vi "PI_Image_Scanner_Prepare.vi"(0 "x-Pixel":u16=100, 1 "y-Pixel":u16=100, 3 "Picture size x":dbl=20.0 min=0.1 max=200.0 format="%1.1f um", 4 "Picture size y":dbl=20.0 min=0.1 max=200.0 format="%1.1f um", 7 "Axis":enum32{"x-y", "x-z", "y-z"}(ring), 9 "Scanner Divider":i32) -> (14 "Commandset out":string[](array[string]), 16 "Measurement time / [s]":dbl)   [LabVIEW 2011]
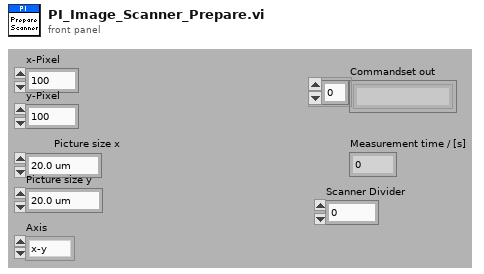
[diagram p1: front panel]
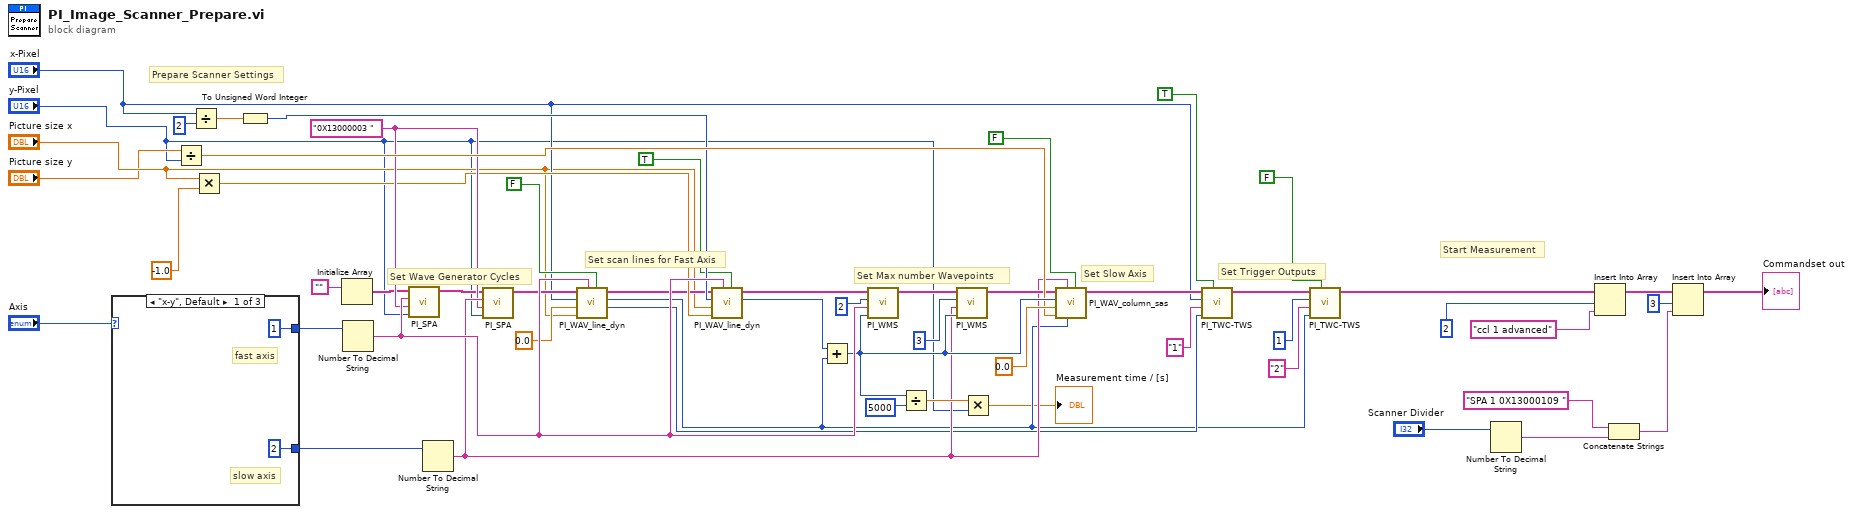
[diagram p0: block diagram]
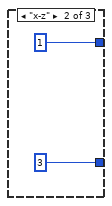
[diagram p2: hidden frame]
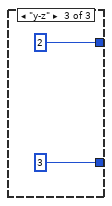
[diagram p3: hidden frame]
diagram:
  w41 = "0X13000003 " ("string")
  # "Start Measurement"
  # "Set Slow Axis"
  # "Set Trigger Outputs"
  # "Set Max number Wavepoints"
  # "Set scan lines for Fast Axis"
  # "Set Wave Generator Cycles"
  # "Prepare Scanner Settings"
  n1 = case shown="\"x-y\", Default" "Axis" {
    tunnel: [1 1 2] -> w27
    tunnel: [2 3 3] -> w28
    frame "x-y", Default {
      # "slow axis"
      # "fast axis"
    }
    frame "x-z" {
    }
    frame "y-z" {
    }
  }
  n2 = Divide(x="Picture size y", y="y-Pixel") -> (x/y=w49:dbl)
  n3 = Divide(x="x-Pixel", y=u16 2) -> (x/y=w33:dbl)
  n4 = Multiply(x="Picture size x", y=-1.0) -> (x*y=w35:dbl)
  n5 = To Unsigned Word Integer(number=w33) -> (unsigned 16bit integer=w34:u16)
  n6 = Initialize Array("") -> (w39:string[])  [unwired: 1 out]
  n7 = Number To Decimal String(number=w27) -> (decimal integer string=w55:string)  [unwired: 1 out]
  n8 = call "PI_SPA.vi"("Value"="y-Pixel", "Register"=w41, "Axis"=w55, "Commandset in"=w39) -> ("Commandset out"=w40:string[])  [unwired: 7 out]
  n9 = Number To Decimal String(number=w28) -> (decimal integer string=w47:string)  [unwired: 1 out]
  n10 = call "PI_SPA.vi"("Value"="y-Pixel", "Register"=w41, "Axis"=w47, "Commandset in"=w40) -> ("Commandset out"=w38:string[])  [unwired: 7 out]
  n11 = call "PI_WAV_line_dyn.vi"("Attach to wav"=FALSE, "Axis Identifier"=w55, "Amplitude / [mu]"="Picture size x", "Startpos / [mu]"=0.0, "Pixel per scan"="x-Pixel", "Commandset in"=w38) -> ("Curve-Start-Pixel"=w24:u16, "Num_Pix"=w17:u16, "Commandset out"=w30:string[])  [unwired: 3 out]
  n12 = call "PI_WAV_line_dyn.vi"("Attach to wav"=TRUE, "Axis Identifier"=w55, "Amplitude / [mu]"=w35, "Startpos / [mu]"="Picture size x", "Pixel per scan"=w34, "Commandset in"=w30) -> ("Num_Pix"=w37:u16, "Commandset out"=w42:string[])  [unwired: 4 out]
  n13 = Add(x=w37, y=w17) -> (x+y=w52:u16)
  n14 = call "PI_WMS.vi"("Pixels to reserve"=w52, "Axis"=w55, "Position / Commandset"=2, "Commandset in"=w42) -> ("Commandset out"=w43:string[])  [unwired: 7 out]
  n15 = Divide(x=w52, y=5000) -> (x/y=w54:dbl)
  n16 = call "PI_WMS.vi"("Pixels to reserve"=w52, "Axis"=w47, "Position / Commandset"=3, "Commandset in"=w43) -> ("Commandset out"=w48:string[])  [unwired: 7 out]
  n17 = Multiply(x=w54, y="y-Pixel") -> (x*y=→"Measurement time / [s]":dbl)
  n18 = call "PI_WAV_column_sas.vi"("Attach to wav"=FALSE, "Steps per Scan-line"=w17, "Axis Identifier"=w47, "Amplitude / [mu]"=w49, "Startpos / [mu]"=0.0, "Pixel per scan"=w52, "Commandset in"=w48) -> ("Commandset out"=w25:string[])  [unwired: 4 out]
  n19 = call "PI_TWC-TWS.vi"("TWC?"=TRUE, "Curve_Start_Pixel"=w24, "Axis Identifier"="1", "Pixel per scan"="x-Pixel", "Commandset in"=w25) -> ("Commandset out"=w21:string[])  [unwired: 6 out]
  n20 = call "PI_TWC-TWS.vi"("TWC?"=FALSE, "Curve_Start_Pixel"=w17, "Axis Identifier"="2", "Pixel per scan"=u16 1, "Commandset in"=w21) -> ("Commandset out"=w5:string[])  [unwired: 6 out]
  n21 = Number To Decimal String(number="Scanner Divider") -> (decimal integer string=w6:string)  [unwired: 1 in]
  n22 = Insert Into Array(array=w5, index=2, new element="ccl 1 advanced" ("Neues Element/Teil-Array")) -> (w12:string[])
  n23 = Concatenate Strings("SPA 1 0X13000109 " ("Neues Element/Teil-Array"), w6) -> (w7:string)
  n24 = Insert Into Array(array=w12, index=3, new element=w7) -> (→"Commandset out":string[])
